vi "Fault Handling.vi"(8 "error in (no error)":errorcluster, 10 "FaultCode":i32, 11 "TestExec in":refnum<class "TestExec.lvclass">) -> (0 "error out":errorcluster, 2 "Fault codes":cluster{"Bit":string, "Description":string}[](array[cluster]), 3 "TestExec out":refnum<class "TestExec.lvclass">)   [LabVIEW 2021, in "OPC UA.lvlib" / "TestExec.lvclass"]
uses:
  TestExec.lvclass
  TestExec.lvclass/TestExec.ctl
  <vilib>/addons/TestStand/_TSUtility.llb/TestStand - Set Property Value (String).vi
  <vilib>/addons/TestStand/_TSUtility.llb/TestStand - Set Property Value (Boolean).vi
  <vilib>/addons/TestStand/_TSUtility.llb/TestStand - Set Property Value (Number).vi
  OPC UA/OPC UA.lvclass
  C:/GitHub/OOP_Submodule EOL/Sequence/CodeModules/OPC UA Client/OPC UA/OPC UA.lvclass
  C:/GitHub/OOP_Submodule EOL/Sequence/CodeModules/OPC UA Client/TestExec/TestExec.lvclass
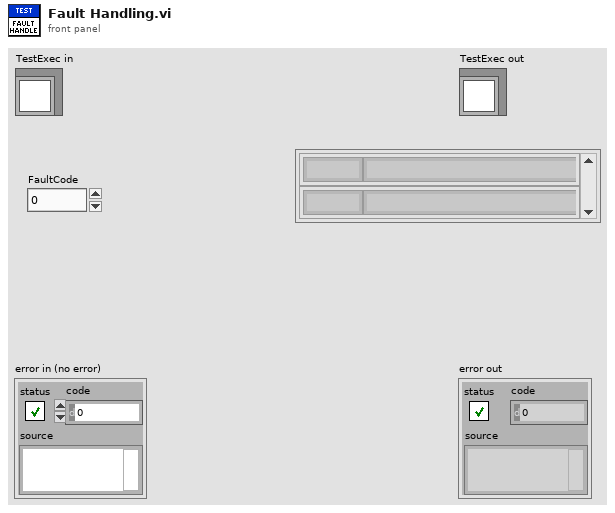
[diagram p1: front panel]
types:
  T1 = typedef "TestExec.lvclass/Rx TestExec.ctl" = cluster{"Cylinder_1":bool, "Cylinder_2":bool, "Cylinder_3":bool, "Cylinder_4":bool, "Cylinder_5":bool, "StepEcho":u32, "Reset":bool, "Stop":bool, "FaultCode":u32}
  T2 = typedef "TestExec.lvclass/Tx TestExec.ctl" = cluster{"HighVoltage":bool, "TestRunning":bool, "StepNo":u32, "Fault":bool}
  T3 = cluster{"FaultCode":i32, "Fault codes":cluster{"Bit":string, "Description":string}[]}
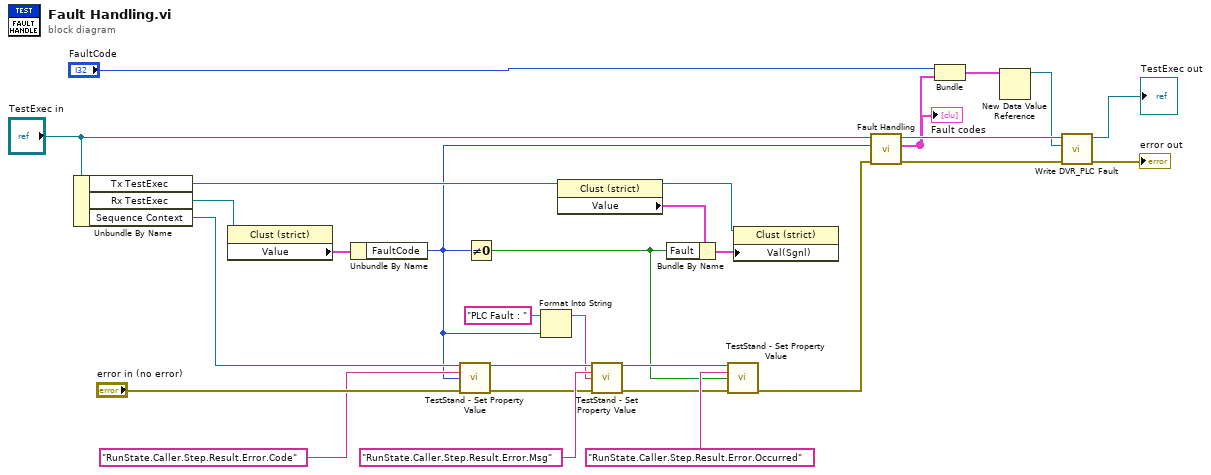
[diagram p0: block diagram]
diagram:
  n1 = Unbundle By Name("TestExec in") -> ("Tx TestExec"=w26:refnum<vi>, "Rx TestExec"=w24:refnum<vi>, "Sequence Context"=w20:refnum<k7>)
  n2 = property class="Clust (strict)"(reference=w24) -> ("Value"=w25:T1)  [unwired: 1 in, 2 out]
  n3 = Unbundle By Name(w25) -> ("FaultCode"=w11:u32)
  n4 = call-poly <vilib>:"TestStand - Set Property Value.vi"("Sequence Context In"=w20, "Lookup String"="RunState.Caller.Step.Result.Error.Code", "New Value"=w11, "error in (no error)"="error in (no error)") -> ("Sequence Context Out"=w15:refnum<k7>, "error out"=w17:errorcluster)  [unwired: 10 in]
  n5 = Not Equal To 0?(x=w11) -> (x != 0?=w9:bool)
  n6 = Format Into String(initial string="PLC Fault : ", w11) -> (resulting string=w12:string)  [unwired: 2 in, 1 out]
  n7 = property class="Clust (strict)"(reference=w26) -> (reference out=w29:refnum<vi>, "Value"=w27:T2)  [unwired: 1 in, 1 out]
  n8 = call-poly <vilib>:"TestStand - Set Property Value.vi"("Sequence Context In"=w15, "Lookup String"="RunState.Caller.Step.Result.Error.Msg", "New Value"=w12, "error in (no error)"=w17) -> ("Sequence Context Out"=w14:refnum<k7>, "error out"=w16:errorcluster)  [unwired: 10 in]
  n9 = Bundle By Name(cluster=w27, "Fault"=w9) -> (w28:T2)
  n10 = call-poly <vilib>:"TestStand - Set Property Value.vi"("Sequence Context In"=w14, "Lookup String"="RunState.Caller.Step.Result.Error.Occurred", "New Value"=w9, "error in (no error)"=w16) -> ("error out"=w10:errorcluster)  [unwired: 10 in, 1 out]
  n11 = property class="Clust (strict)"(reference=w29, "Val(Sgnl)"=w28) -> ()  [unwired: 1 in, 2 out]
  n12 = call-parent "Fault Handling.vi"("error in (no error)"=w10, "FaultCode"=w11, "OPC UA in"="TestExec in") -> ("error out"=w5:errorcluster, "Fault codes"=w3:cluster{"Bit":string, "Description":string}[], "OPC UA out"=w7:refnum<class "TestExec.lvclass">)  [unwired: 6 in]
  "Fault codes" <- w3
  n13 = Bundle("FaultCode"="FaultCode", "Fault codes"=w3) -> (w2:T3)  [unwired: 1 in]
  n14 = New Data Value Reference(data value=w2) -> (data value reference=w1:refnum<data-value>)  [unwired: 1 in, 1 out]
  n15 = call "Write DVR_PLC Fault.vi"("error in (no error)"=w5, "DVR_PLC Fault"=w1, "OPC UA in"=w7) -> ("error out"=→"error out":errorcluster, "OPC UA out"=→"TestExec out":refnum<class "TestExec.lvclass">)  [unwired: 7 in]
